vi "SVT UFF58 Read Records 1 to 3.vi"(0 "function refnum":refnum<k20>, 11 "error in (no error)":errorcluster) -> (4 "dup function refnum":refnum<k20>, 6 "ID lines (1-3)":T1, 15 "error out":errorcluster)   [LabVIEW 2017, in "SoundVib_UFF58.lvlib"]
doc: "Reads the values of records 1, 2, and 3 of a UFF58 (universal file format) file. Record 1 typically is used for the function description. Record 3 typically is used to identify when the function was created."
uses:
  <vilib>/addons/Sound and Vibration/svt_UFF58/SoundVib_UFF58.lvlib
  <vilib>/addons/Sound and Vibration/svt_UFF58/subVIs/sv_IDLines123.ctl
  <vilib>/Platform/storage/Storage.llb/Get Property (String).vi
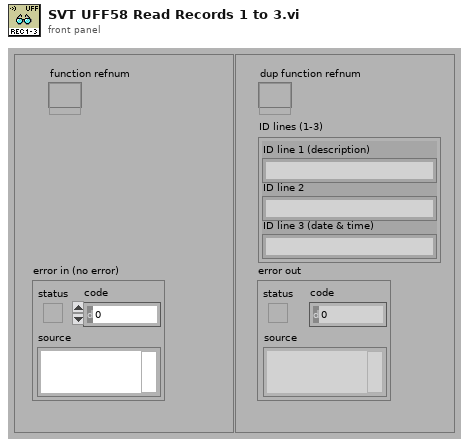
[diagram p1: front panel]
types:
  T1 = typedef "SoundVib_UFF58.lvlib/sv_IDLines123.ctl" = cluster{"ID line 1 (description)":string, "ID line 2":string, "ID line 3 (date & time)":string}
  T2 = cluster{"output string":string, "output string":string, "output string":string}
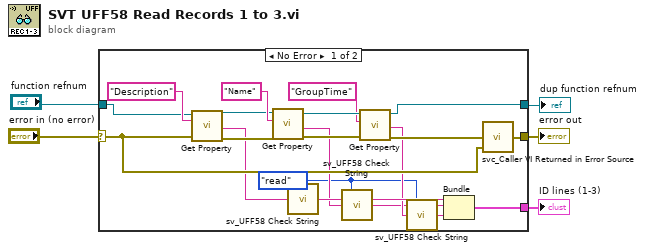
[diagram p0: block diagram]
diagram:
  n1 = case shown="No Error" "error in (no error)" {
    selector: "error in (no error)" -> [w13 w26]
    tunnel: [w24 _] -> w5
    tunnel: "function refnum" -> [w22 w27]
    tunnel: [w19 w27] -> w1
    tunnel: [w14 w26] -> w4
    frame No Error {
      w6 = enum16{"read", "write"}."read" ("operation")
      n2 = call-poly <vilib>:"Get Property.vi"("error in (no error)"=w13, "Property name"="Description", "storage refnum"=w22) -> ("error out"=w20:errorcluster, "Value"=w12:string, "storage refnum out"=w21:refnum<k20>)  [unwired: 6 in]
      n3 = call-poly <vilib>:"Get Property.vi"("error in (no error)"=w20, "Property name"="Name", "storage refnum"=w21) -> ("error out"=w18:errorcluster, "Value"=w8:string, "storage refnum out"=w17:refnum<k20>)  [unwired: 6 in]
      n4 = call <vilib>:"sv_UFF58 Check String.vi"("operation"=w6, "field value"=w12) -> ("output string"=w11:string)  [unwired: 12 in, 1 out]
      n5 = call <vilib>:"sv_UFF58 Check String.vi"("operation"=w6, "field value"=w8) -> ("output string"=w7:string)  [unwired: 12 in, 1 out]
      n6 = call-poly <vilib>:"Get Property.vi"("error in (no error)"=w18, "Property name"="GroupTime", "storage refnum"=w17) -> ("error out"=w15:errorcluster, "Value"=w9:string, "storage refnum out"=w19:refnum<k20>)  [unwired: 6 in]
      n7 = call <vilib>:"sv_UFF58 Check String.vi"("operation"=w6, "field value"=w9) -> ("output string"=w10:string)  [unwired: 12 in, 1 out]
      n8 = Bundle("output string"=w11, "output string"=w7, "output string"=w10) -> (w24:T2)  [unwired: 1 in]
      n9 = call <vilib>:"svc_Caller VI Returned in Error Source.vi"("warning input to caller"=w13, "error in (no error)"=w15) -> ("error out"=w14:errorcluster)  [unwired: 3 in]
    }
    frame Error {
    }
  }
  "error out" <- w4
  "ID lines (1-3)" <- w5
  "dup function refnum" <- w1
